vi "Framework Status.Set Performance.vi"(10 "Framework Performance":refnum<class "Framework Performance.lvclass">, 11 "Framework Status in":refnum<class "Framework Status.lvclass">) -> (3 "Framework Status out":refnum<class "Framework Status.lvclass">)   [LabVIEW 2017, in "DSF Core.lvlib" / "Framework Status.lvclass"]
uses:
  Framework Status.lvclass
  Framework Performance.lvclass
  Framework Status.lvclass/Framework Status.ctl
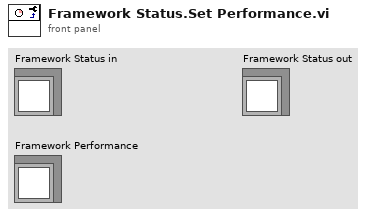
[diagram p1: front panel]
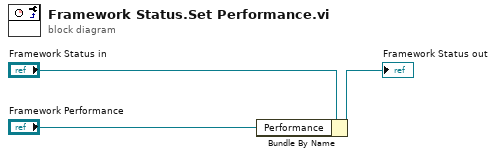
[diagram p0: block diagram]
diagram:
  n1 = Bundle By Name(cluster="Framework Status in", "Performance"="Framework Performance") -> (→"Framework Status out":refnum<class "Framework Status.lvclass">)
